vi "checkForILCTimeouts.vi"(8 "error in (no error)":errorcluster, 11 "Model in":refnum<class "Model.lvclass">) -> (0 "error out":errorcluster, 3 "Model out":refnum<class "Model.lvclass">)   [LabVIEW 2016, in "Model.lvclass"]
uses:
  Model.lvclass
  Model.lvclass/Model.ctl
  ILCCommunications/ILCCommunications.lvclass
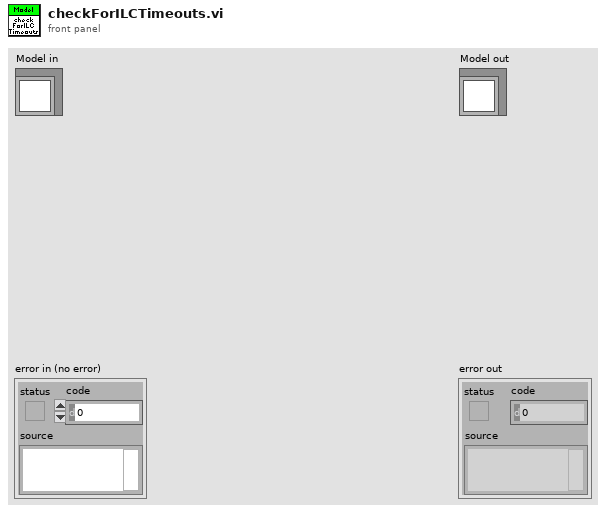
[diagram p1: front panel]
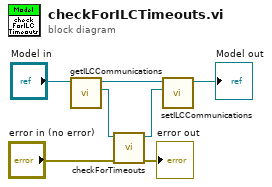
[diagram p0: block diagram]
diagram:
  n1 = call "getILCCommunications.vi"("Model in"="Model in") -> ("ILCCommunications"=w5:refnum<class "ILCCommunications.lvclass">, "Model out"=w7:refnum<class "Model.lvclass">)  [unwired: 9 in]
  n2 = call "checkForTimeouts.vi"("error in (no error)"="error in (no error)", "ILCCommunications in"=w5) -> ("error out"=→"error out":errorcluster, "ILCCommunications out"=w6:refnum<class "ILCCommunications.lvclass">)  [unwired: 8 in]
  n3 = call "setILCCommunications.vi"("ILCCommunications"=w6, "Model in"=w7) -> ("Model out"=→"Model out":refnum<class "Model.lvclass">)  [unwired: 9 in]
